vi "Teleop_Joystick Deadband.vi"(9 "Joystick %Linear":dbl[](array[numeric])=[0.5, 0.5, 0.5, 1.0] format="%.2f", 10 "Joystick Deadbands":dbl[](array[numeric])=[0.1, 0.1, 0.1, 0.0] format="%.2f", 11 "Joystick Axes in":dbl[](array[numeric])=[0.0, 0.0, 0.0, 0.0] format="%.2f") -> (3 "Joystick Axes out":dbl[](array[numeric])=[-3.009265538105056e-32, 0.0, 0.0, 0.0] format="%.2f")   [LabVIEW 2016]
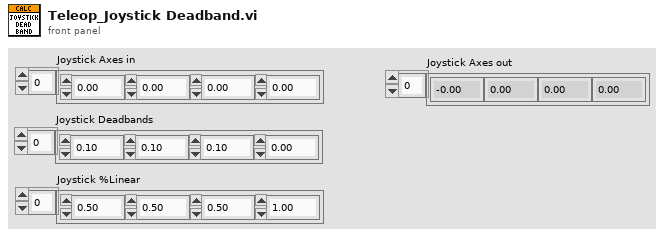
[diagram p1: front panel]
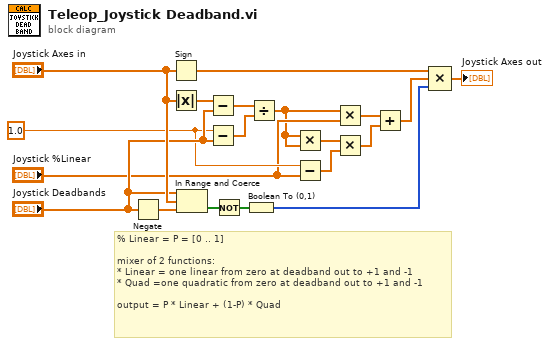
[diagram p0: block diagram]
diagram:
  w9 = 1.0
  # "% Linear = P = [0 .. 1]\n\nmixer of 2 functions:\n* Linear = one linear from zero at deadband out to +1 and -1\n* Quad =one quadratic from zero at deadband out to +1 and -1\n\noutput = P * Linear + (1-P) * Quad"
  n1 = Negate(x="Joystick Deadbands") -> (-x=w19:dbl[])
  n2 = Sign(1:"Joystick Axes in") -> (0:w2:dbl[])
  n3 = Absolute Value(x="Joystick Axes in") -> (abs(x)=w13:dbl[])
  n4 = In Range and Coerce(upper limit="Joystick Deadbands", x="Joystick Axes in", lower limit=w19) -> (In Range?=w18:bool[])  [unwired: 1 out]
  n5 = Subtract(x=w13, y="Joystick Deadbands") -> (x-y=w12:dbl[])
  n6 = Subtract(x=w9, y="Joystick Deadbands") -> (x-y=w10:dbl[])
  n7 = Not(x=w18) -> (.not. x?=w15:bool[])
  n8 = Boolean To (0,1)(Boolean=w15) -> (0, 1=w17:i16[])
  n9 = Divide(x=w12, y=w10) -> (x/y=w7:dbl[])
  n10 = Multiply(x=w7, y=w7) -> (x*y=w6:dbl[])
  n11 = Subtract(x=w9, y="Joystick %Linear") -> (x-y=w5:dbl[])
  n12 = Multiply(x=w7, y="Joystick %Linear") -> (x*y=w4:dbl[])
  n13 = Multiply(x=w6, y=w5) -> (x*y=w3:dbl[])
  n14 = Add(x=w4, y=w3) -> (x+y=w1:dbl[])
  n15 = Compound Arithmetic op=MULTIPLY(w2, w1, w17) -> (→"Joystick Axes out":dbl[])
